vi "Main.vi"   [LabVIEW 2017]
uses:
  Communication/QueueRepo.Action.ctl
  GUI/Main/MainGUI.lvlib
  GUI/DAQConfig/DAQConfig.lvlib
  Communication/Communication.lvlib
  GUI/Chart/Chart.lvlib
  DAQ/DAQ.lvlib
types:
  T1 = enum32{"Invalid", "Standard", "Closed", "Hidden", "Minimized", "Maximized"}
  T2 = typedef "Communication.lvlib/QueueRepo.Action.ctl" = enum16{"Add", "Get", "Destroy", "Get All", "Clear"}
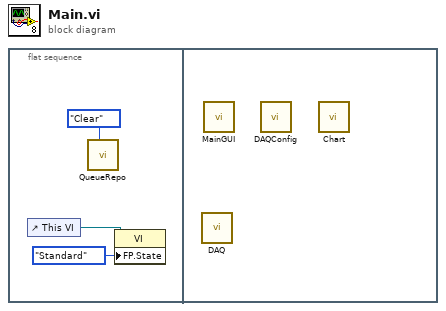
[diagram p0: block diagram]
diagram:
  n1 = flat-sequence {
    frame #0 {
      n2 = control-ref of="This VI"() -> (w2:refnum<vi>)
      n3 = call "QueueRepo.vi"("Action"=QueueRepo.Action."Clear") -> ()  [unwired: 7 in, 4 out]
      n4 = property class="VI"(reference=w2, "FP.State"=T1."Standard" ("Front Panel Window:State")) -> ()  [unwired: 1 in, 2 out]
    }
    frame #1 {
      n5 = call "DAQ.vi"() -> ()  [unwired: 12 in]
      n6 = call "MainGUI.vi"() -> ()  [unwired: 12 in]
      n7 = call "DAQConfig.vi"() -> ()  [unwired: 12 in]
      n8 = call "Chart.vi"() -> ()  [unwired: 12 in]
    }
  }
